vi "Settings Dictionary.vi"(0 "Setting name":string, 1 "Action":T1, 5 "Setting value":string) -> (4 "Setting already included? / Setting not found?":bool, 6 "Setting value out":string)   [LabVIEW 2023, in "RFCalAndFixtureCharact.Common.lvlib"]
uses:
  RFCalAndFixtureCharact.Common.lvlib
  Type Definitions/Dictionary Operation.ctl
  <vilib>/Utility/miscctls.llb/LVMapReplaceAction.ctl
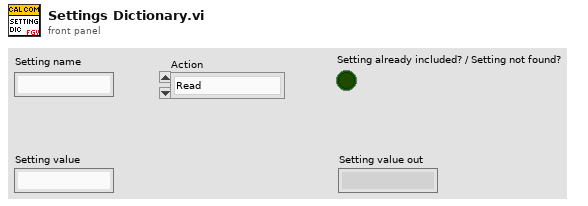
[diagram p1: front panel]
types:
  T1 = typedef "RFCalAndFixtureCharact.Common.lvlib/Dictionary Operation.ctl" = enum16{"Read", "Insert", "Remove", "Clear", "Get All", "Update"}
  T2 = typedef "LVMapReplaceAction.ctl" = enum32{"Modify Entry only if found", "Add or Modify Entry", "Delete Entry"}
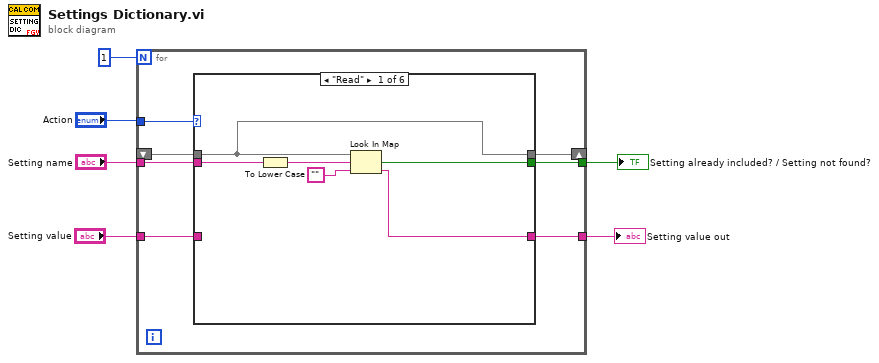
[diagram p0: block diagram]
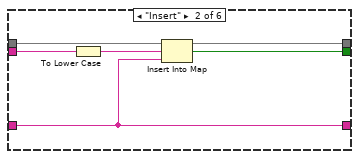
[diagram p2: hidden frame]
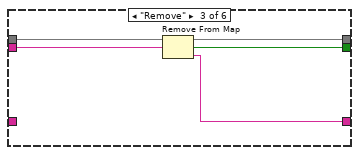
[diagram p3: hidden frame]
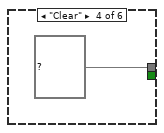
[diagram p4: hidden frame]
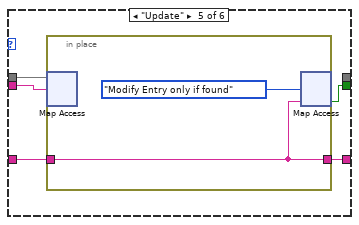
[diagram p5: hidden frame]
diagram:
  n1 = for {
    N: 1 -> [_]
    tunnel: "Action" -> [w13]
    tunnel: "Setting name" -> [w12]
    tunnel: [w11] -> w4
    tunnel: [w10] -> w1
    shift-right: [w7] -> _
    shift-left: _ -> [w9]
    tunnel: "Setting value" -> [w8]
    n2 = case shown="\"Read\"" w13 {
      tunnel: w12 -> [w19 w25 w29 _ w35 _]
      tunnel: w9 -> [w16 w22 w27 _ w36 w40]
      tunnel: [w18 w24 w30 _ w33 _] -> w11
      tunnel: [w17 w23 w28 _ w32 w39] -> w10
      tunnel: w8 -> [_ w23 _ _ w34 w39]
      tunnel: [w16 w21 w26 map{string, string} {} ("map") _ w40] -> w7
      frame "Read" {
        n3 = To Lower Case(string=w19) -> (all lower case string=w14:string)
        n4 = Look In Map(map=w16, key=w14, default value="") -> (key not found?=w18:bool, value=w17:string)
      }
      frame "Insert" {
        n5 = To Lower Case(string=w25) -> (all lower case string=w20:string)
        n6 = Insert Into Map(map in=w22, key=w20, value=w23) -> (map out=w21:map{string, string}, key already included?=w24:bool)  [unwired: 1 out]
      }
      frame "Remove" {
        n7 = Remove From Map(10:w29, 11:w27) -> (1:w28:string, 2:w30:bool, 3:w26:map{string, string})
      }
      frame "Clear" {
      }
      frame "Update" {
        n8 = in-place {
          in-place-border: w34 -> [w37]
          in-place-border: [w37] -> w32
          n9 = in-place-map #1(w36, w35) -> ()  [unwired: 1 in, 2 out]
          n10 = in-place-map #1(w37, LVMapReplaceAction."Modify Entry only if found" ("action")) -> (w33:bool)  [unwired: 2 out]
        }
      }
      frame Default {
      }
    }
  }
  "Setting already included? / Setting not found?" <- w4
  "Setting value out" <- w1
